vi "Rounding Number.vi"(9 "Power of ten":dbl, 10 "Number to round":dbl=1234.56789 format="%_9f") -> (1 "Decimal place":dbl=1.0 format="%#_9f", 2 "Rounded number":dbl=1235.0 format="%_9f")   [LabVIEW 2011]
doc: "LabVIEW only readily supports rounding numbers to integer values. For example, LabVIEW rounds the number 543.21 to 543.00.\n\nThis VI shows how to round numbers to values other than integers. For example, you can round the number 543.21 to 543.20 or 540.00 by choosing which decimal place you want to round to."
panel:
  # "Select Help»Show Context Help and move the cursor over the VI icon to display help for this VI."
  # "Instructions:\n1. Run the VI.\n2. Enter a number you want to round.\n3. Enter a power of ten to select which decimal place to round to.\n4. Repeat steps 2 and 3 until you no longer want to round numbers.\n5. Click the Stop button to stop the VI."
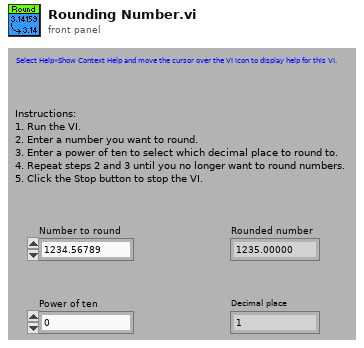
[diagram p1: front panel]
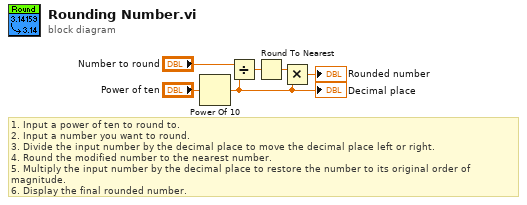
[diagram p0: block diagram]
diagram:
  # "1. Input a power of ten to round to.\n2. Input a number you want to round.\n3. Divide the input number by the decimal place to move the decimal place left or right.\n4. Round the modified number to the nearest number.\n5. Multiply the input number by the decimal place to restore the number to its original order of magnitude.\n6. Display the final rounded number."
  n1 = Power Of 10(x="Power of ten") -> (10^x=w2:dbl)
  "Decimal place" <- w2
  n2 = Divide(x="Number to round", y=w2) -> (x/y=w5:dbl)
  n3 = Round To Nearest(number=w5) -> (nearest integer value=w4:dbl)
  n4 = Multiply(x=w4, y=w2) -> (x*y=→"Rounded number":dbl)
